vi "CAlex2_InitAll_Hv.vi"(8 "error in (no error)":errorcluster, 9 "ExtraWeight(kg)":cluster{"Thigh":dbl, "Shank":dbl}, 10 "LegProperties":T1={"BodyDim(m)"={"ThighLt"=0.4, "ShankLt"=0.41, "HipWd"=0.32}, "BodyWt(kg)"={"Thigh"=0.0, "Shank"=0.0}, "CuffLoc(m)"={"HipCuffWd"=0.4, "HipCuffHt"=0.1, "HipCuffFwdShift"=0.0, "ThighCuffToKnee"=0.25, "ThighCuffDist"=0.0, "ShankCuffToKnee"=0.15}}, 11 "CAlex2 in":refnum<class "CAlex2.lvclass">) -> (0 "error out":errorcluster, 3 "CAlex2 out":refnum<class "CAlex2.lvclass">)   [LabVIEW 2015, in "CAlex2.lvclass"]
uses:
  CAlex2.lvclass
  TypeDef/LowerBodyDim.ctl
  Body/xyzO.ctl
  <vilib>/Analysis/Matrix/Datatypes/RealMatrix.ctl
  CAlex2.lvclass/CAlex2.ctl
  Body/Bodies.lvclass
  <vilib>/Analysis/Matrix/NI_Matrix.lvlib
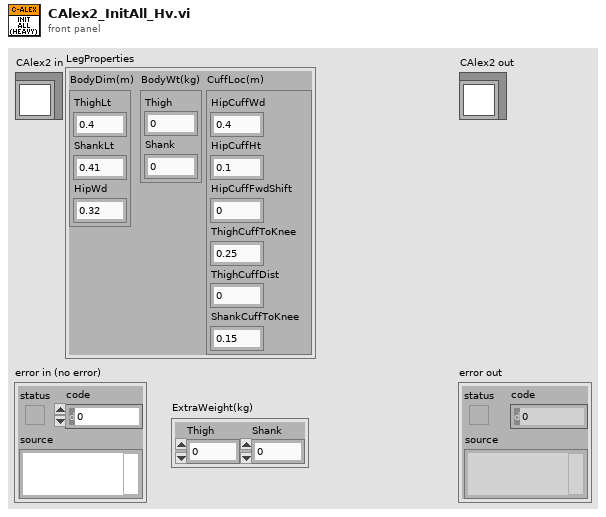
[diagram p1: front panel]
types:
  T1 = typedef "CAlex2.lvclass/LowerBodyDim.ctl" = cluster{"BodyDim(m)":cluster{"ThighLt":dbl, "ShankLt":dbl, "HipWd":dbl}, "BodyWt(kg)":cluster{"Thigh":dbl, "Shank":dbl}, "CuffLoc(m)":cluster{"HipCuffWd":dbl, "HipCuffHt":dbl, "HipCuffFwdShift":dbl, "ThighCuffToKnee":dbl, "ThighCuffDist":dbl, "ShankCuffToKnee":dbl}}
  T2 = typedef "NI_Matrix.lvlib/RealMatrix.ctl" = dbl[][]
  T3 = typedef "Bodies.lvclass/xyzO.ctl" = enum16{"X", "Y", "Z", "O"}
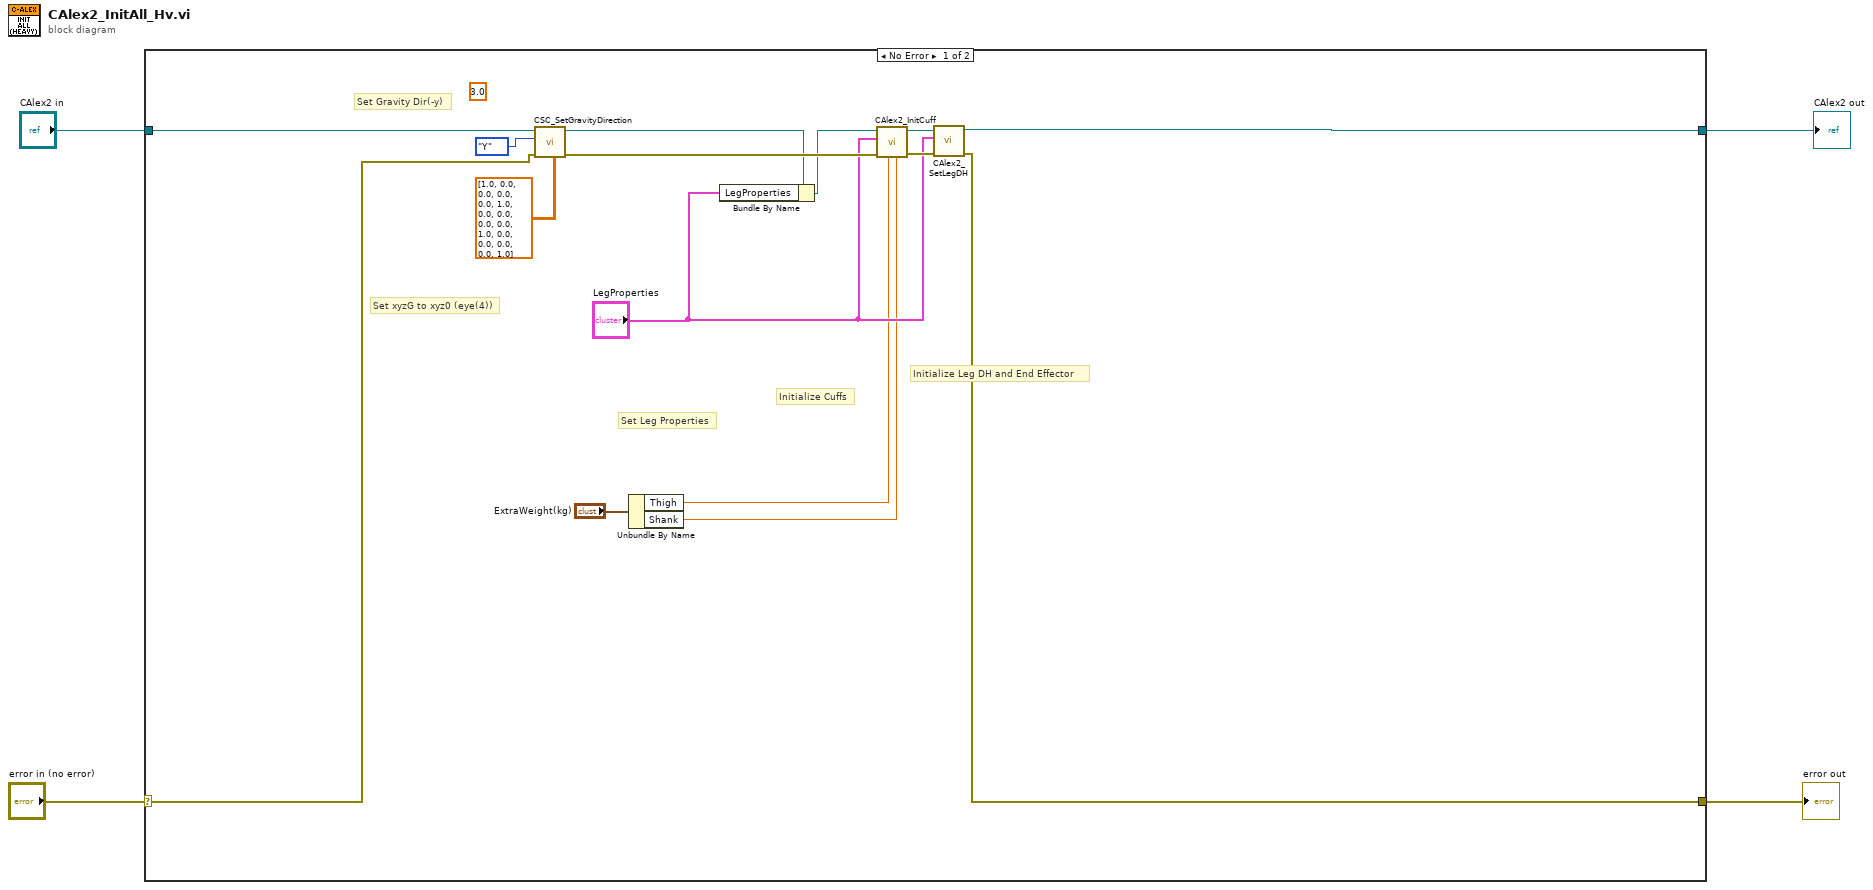
[diagram p0: block diagram]
diagram:
  n1 = case shown="No Error" "error in (no error)" {
    selector: "error in (no error)" -> [w10 w21]
    tunnel: [w9 w21] -> w3
    tunnel: [w16 w20] -> w1
    tunnel: "CAlex2 in" -> [w18 w20]
    frame No Error {
      (unwired) 3.0 ("Numeric")
      # "Initialize Leg DH and End Effector"
      # "Initialize Cuffs"
      # "Set Leg Properties"
      # "Set xyzG to xyz0 (eye(4))"
      # "Set Gravity Dir(-y)"
      n2 = call-dynamic "CSC_SetGravityDirection.vi"("Trans_Gto0"=T2 [[1.0, 0.0, 0.0, 0.0], [0.0, 1.0, 0.0, 0.0], [0.0, 0.0, 1.0, 0.0], [0.0, 0.0, 0.0, 1.0]] ("Trans_0toG"), "error in (no error)"=w10, "Gravity Axis in G (Z)"=xyzO."Y" ("Gravity Axis"), "CSC in"=w18) -> ("error out"=w14:errorcluster, "CSC out"=w13:refnum<class "CAlex2.lvclass">)  [unwired: 6 in]
      n3 = Unbundle By Name("ExtraWeight(kg)") -> ("Thigh"=w6:dbl, "Shank"=w5:dbl)
      n4 = Bundle By Name(cluster=w13, "LegProperties"="LegProperties") -> (w11:refnum<class "CAlex2.lvclass">)
      n5 = call-dynamic "CAlex2_InitCuff.vi"("ShankExtraWeight"=w5, "ThighExtraWeight"=w6, "error in (no error)"=w14, "LegProperty"="LegProperties", "CAlex2 in"=w11) -> ("error out"=w15:errorcluster, "CAlex2 out"=w17:refnum<class "CAlex2.lvclass">)  [unwired: 5 in]
      n6 = call-dynamic "CAlex2_SetLegDH.vi"("error in (no error)"=w15, "ArmProperty"="LegProperties", "CAlex2 in"=w17) -> ("error out"=w9:errorcluster, "CAlex2 out"=w16:refnum<class "CAlex2.lvclass">)  [unwired: 7 in]
    }
    frame Error {
    }
  }
  "error out" <- w3
  "CAlex2 out" <- w1
